vi "Check - Unique QControl Name.vi"(11 "New QControl Info":refnum<data-value>) -> (0 "error out":errorcluster)   [LabVIEW 2020, in "New QControl Info.lvclass"]
doc: "<b> </b> <b> </b>\n©2016 Q Software Innovations, LLC (QSI)\nwritten by Quentin Alldredge\nproduced in LabVIEW 2015\n\nsupport@qsoftwareinnovations.com\nwww.qsoftwareinnovations.com\n\nAll rights reserved.\n\nRedistribution and use in source and binary forms, with or without modification, are permitted provided that the following conditions are met:\n\n * Redistributions of source code must retain the above copyright notice, this list of conditions and the following disclaimer.\n * Redistributions in binary form must reproduce the above copyright notice, this list of conditions and the following disclaimer in the documentation and/or other materials provided with the distribution.\n * Neither the name of Q Software Innovations, LLC. nor the names of its contributors may be used to endorse or promote products derived from this software without specific prior written permission.\n\nTHIS SOFTWARE IS PROVIDED BY THE COPYRIGHT HOLDERS AND CONTRIBUTORS \"AS IS\" AND ANY EXPRESS OR IMPLIED WARRANTIES, INCLUDING, BUT NOT LIMITED TO, THE IMPLIED WARRANTIES OF MERCHANTABILITY AND FITNESS FOR A PARTICULAR PURPOSE ARE DISCLAIMED. IN NO EVENT SHALL THE COPYRIGHT OWNER OR CONTRIBUTORS BE LIABLE FOR ANY DIRECT, INDIRECT, INCIDENTAL, SPECIAL, EXEMPLARY, OR CONSEQUENTIAL DAMAGES (INCLUDING, BUT NOT LIMITED TO, PROCUREMENT OF SUBSTITUTE GOODS OR SERVICES; LOSS OF USE, DATA, OR PROFITS; OR BUSINESS INTERRUPTION) HOWEVER CAUSED AND ON ANY THEORY OF LIABILITY, WHETHER IN CONTRACT, STRICT LIABILITY, OR TORT (INCLUDING NEGLIGENCE OR OTHERWISE) ARISING IN ANY WAY OUT OF THE USE OF THIS SOFTWARE, EVEN IF ADVISED OF THE POSSIBILITY OF SUCH DAMAGE."
uses:
  New QControl Info/New QControl Info.lvclass
  QControl Classes/Control/Control.lvclass
  New QControl Info/New QControl Info.lvclass/New QControl Info.ctl
  New QControl Info/Read New Class Path.vi
  <vilib>/ErrorRing/Error Ring.xnode
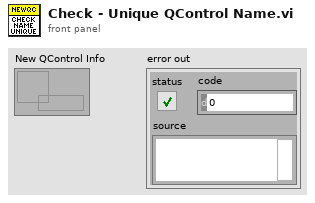
[diagram p1: front panel]
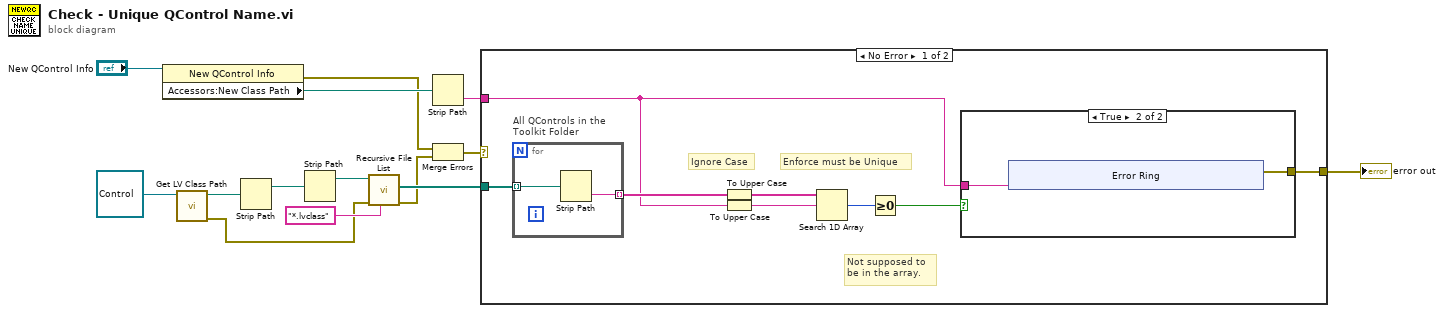
[diagram p0: block diagram]
diagram:
  n1 = property class="New QControl Info"(reference="New QControl Info") -> (error out=w4:errorcluster, "Accessors:New Class Path"=w6:path)  [unwired: 1 in, 1 out]
  n2 = call <vilib>:"Get LV Class Path.vi"("object"=refnum<class "Control.lvclass"> refnum ("Control")) -> ("error out"=w5:errorcluster, "class path"=w10:path)  [unwired: 9 in]
  n3 = Strip Path(path=w10) -> (stripped path=w9:path)  [unwired: 1 out]
  n4 = Strip Path(path=w9) -> (stripped path=w11:path)  [unwired: 1 out]
  n5 = call <vilib>:"Recursive File List.vi"("pattern"="*.lvclass", "error in (no error)"=w5, "Folder Path"=w11) -> ("error out"=w3:errorcluster, "All Files in Dir"=w14:path[])  [unwired: 4 in, 3 out]
  n6 = Strip Path(path=w6) -> (name=w1:string)  [unwired: 1 out]
  n7 = Merge Errors(w4, w3) -> (w2:errorcluster)
  n8 = case shown="No Error" w2 {
    selector: w2 -> [_ w32]
    tunnel: w14 -> [w18 _]
    tunnel: [w16 w32] -> w8
    tunnel: w1 -> [w15 _]
    frame No Error {
      # "Not supposed to\nbe in the array."
      # "Ignore Case"
      # "Enforce must be Unique"
      n9 = for "All QControls in the \nToolkit Folder" {
        tunnel: w18 -> [w31] mode=indexing
        tunnel: [w30] -> w22 mode=indexing
        n10 = Strip Path(path=w31) -> (name=w30:string)  [unwired: 1 out]
      }
      n11 = To Upper Case(1:w22) -> (0:w20:string[])
      n12 = To Upper Case(1:w15) -> (0:w19:string)
      n13 = Search 1D Array(1D array=w20, element=w19) -> (index of element=w21:i32)  [unwired: 1 in]
      n14 = Greater Or Equal To 0?(x=w21) -> (x >= 0?=w17:bool)
      n15 = case shown="True" w17 {
        tunnel: w15 -> [_ w24]
        tunnel: [_ w23] -> w16
        frame False {
        }
        frame True {
          n16 = xnode "Error Ring"("parameter 0"=w24) -> ("error out"=w23:errorcluster)
        }
      }
    }
    frame Error {
    }
  }
  "error out" <- w8
